vi "get working area.vi"(8 "error in (no error)":errorcluster) -> (0 "error out":errorcluster, 3 "screens":T1[](array[typedef]))   [LabVIEW 2021, in "TipStripOOPanel.lvlib"]
uses:
  TipStripOOPanel.lvlib
  tipstrip_screens.ctl
  System.Windows.Forms
  System.Drawing
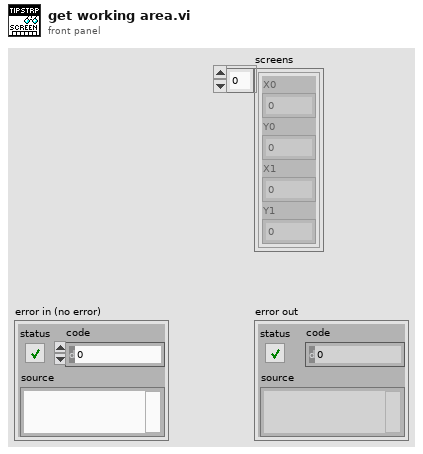
[diagram p1: front panel]
types:
  T1 = typedef "TipStripOOPanel.lvlib/tipstrip_screens.ctl" = cluster{"X0":i32, "Y0":i32, "X1":i32, "Y1":i32}
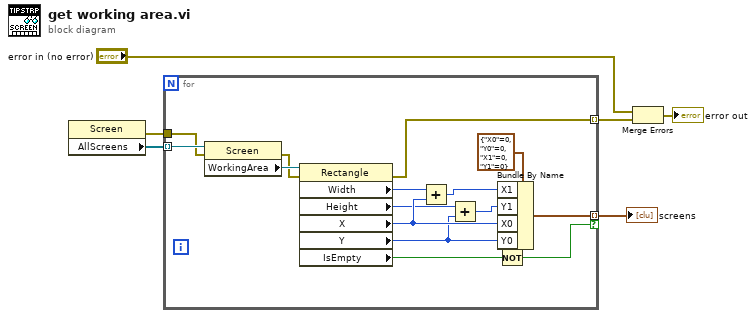
[diagram p0: block diagram]
diagram:
  n1 = property class="Screen"() -> (error out=w5:errorcluster, "AllScreens"=w6:refnum<k24>[])  [unwired: 2 in, 1 out]
  n2 = for {
    tunnel: w6 -> [w21] mode=indexing
    tunnel: w5 -> [w19]
    tunnel: [w16] -> w4 mode=indexing if=w14
    tunnel: [w7] -> w3 mode=indexing
    n3 = property class="Screen"(reference=w21, error in=w19) -> (error out=w18:errorcluster, "WorkingArea"=w20:refnum<k24>)  [unwired: 1 out]
    n4 = property class="Rectangle"(reference=w20, error in=w18) -> (error out=w7:errorcluster, "Width"=w13:i32, "Height"=w10:i32, "X"=w12:i32, "Y"=w9:i32, "IsEmpty"=w15:bool)  [unwired: 1 out]
    n5 = Add(x=w13, y=w12) -> (x+y=w11:i32)
    n6 = Add(x=w10, y=w9) -> (x+y=w8:i32)
    n7 = Not(x=w15) -> (.not. x?=w14:bool)
    n8 = Bundle By Name(cluster=T1 {"X0"=0, "Y0"=0, "X1"=0, "Y1"=0}, "X1"=w11, "Y1"=w8, "X0"=w12, "Y0"=w9) -> (w16:T1)
  }
  "screens" <- w4
  n9 = Merge Errors("error in (no error)", w3) -> (→"error out":errorcluster)
